vi "SIRCenterStripHole.vi"(7 "center hole":dbl format="%.2f", 8 "P":cluster{"x":dbl, "y":dbl, "z":dbl}={"x"=1.0, "y"=-5.0, "z"=1.0} {"x" format="%.2f"; "z" format="%.2f"; "y" format="%.2f"}, 9 "Variables":T1={"sound spd (cm/s)"=150000, "time step (s)"=1e-09} {"time step (s)" format="%.2e"}, 11 "strip":cluster{"Radius":dbl, "h":dbl, "a":dbl}={"Radius"=10.0, "h"=3.0, "a"=5.0} {"Radius" format="%.2f"; "a" format="%.2f"; "h" format="%.2f"}) -> (1 "lower":dbl[](graph), 2 "upper":dbl[](graph), 3 "h out":dbl[](graph), 4 "delay out":i32)   [LabVIEW 2022 SP3]
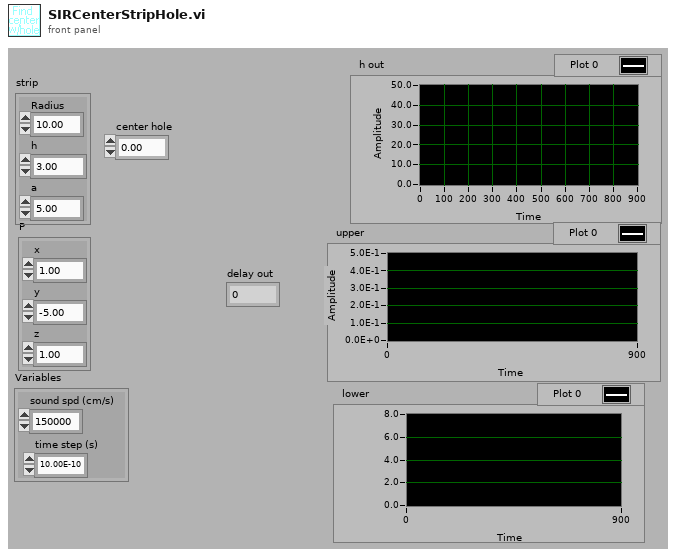
[diagram p1: front panel]
types:
  T1 = cluster{"sound spd (cm/s)":i32, "time step (s)":sgl}
  T2 = cluster{"Number of rings":i32, "sound spd (cm/s)":i32, "z span (cm)":dbl, "z steps":i32, "y span (cm)":dbl, "y steps":i32, "time step (s)":sgl, "z":dbl, "y":dbl, "ref delay":dbl, "freq (MHz)":dbl, "cycles":i32}
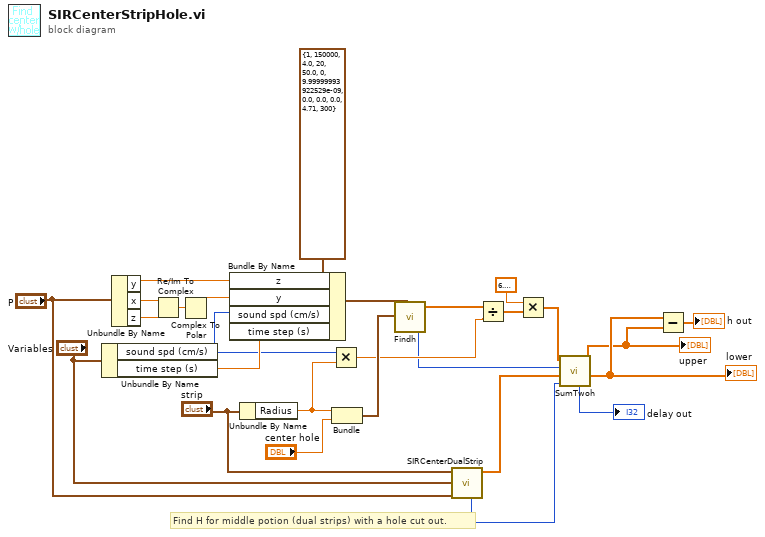
[diagram p0: block diagram]
diagram:
  # "Find H for middle potion (dual strips) with a hole cut out."
  n1 = Unbundle By Name("Variables") -> ("sound spd (cm/s)"=w20:i32, "time step (s)"=w23:sgl)
  n2 = Unbundle By Name("P") -> ("y"=w21:dbl, "x"=w26:dbl, "z"=w25:dbl)
  n3 = Re/Im To Complex(1:w25, 2:w26) -> (0:w24:cdb)
  n4 = Complex To Polar(r * e^(i*theta)=w24) -> (r=w22:dbl)  [unwired: 1 out]
  n5 = Bundle By Name(cluster=T2 {"Number of rings"=1, "sound spd (cm/s)"=150000, "z span (cm)"=4.0, "z steps"=20, "y span (cm)"=50.0, "y steps"=0, "time step (s)"=1e-08, "z"=0.0, "y"=0.0, "ref delay"=0.0, "freq (MHz)"=4.71, "cycles"=300} ("Variables in"), "z"=w21, "y"=w22, "sound spd (cm/s)"=w20, "time step (s)"=w23) -> (w16:T2)
  n6 = Unbundle By Name("strip") -> ("Radius"=w3:dbl)
  n7 = Multiply(x=w20, y=w3) -> (x*y=w10:dbl)
  n8 = Bundle("Radius"=w3, "center hole"="center hole") -> (w14:cluster{"Radius":dbl, "center hole":dbl})  [unwired: 1 out]
  n9 = call "Findh.vi"("Trans Geometry"=w14, "Variables in"=w16) -> ("h(r,t)"=w11:dbl[], "delay pts"=w9:i32)  [unwired: 1 in, 3 out]
  n10 = call "SIRCenterDualStrip.vi"("P"="P", "Variables"="Variables", "strip"="strip") -> ("h out"=w1:dbl[], "delay out"=w8:i32)  [unwired: 7 out]
  n11 = Divide(x=w11, y=w10) -> (x/y=w13:dbl[])
  n12 = Multiply(x=6.283185307179586, y=w13) -> (x*y=w2:dbl[])
  n13 = call "SumTwoh.vi"("h1"=w2, "delay1"=w9, "h2"=w1, "delay2"=w8) -> ("delay out"=→"delay out":i32, "upper"=w6:dbl[], "lower"=w7:dbl[])  [unwired: 2 out]
  "upper" <- w6
  "lower" <- w7
  n14 = Subtract(x=w7, y=w6) -> (x-y=→"h out":dbl[])
